vi "Begin.vi"() -> (0 "error out":errorcluster)   [LabVIEW 2011]
doc: "Called before other user functions, this VI is expected to open initial I/O refnums, load in file data, and do all program initialization. Notice that the <B>error out</B> terminal is simply used for data flow. Wiring it to other structures or subVIs ensures that this VI runs first."
uses:
  <vilib>/Rock Robotics/WPI/Joystick/WPI_JoystickDeviceEnum.ctl
  <vilib>/Rock Robotics/SystemInterfaces/DIO/FPGA_DIOPWMChannel.ctl
  <vilib>/Rock Robotics/SystemInterfaces/DIO/FPGA_DIOChannel.ctl
  <vilib>/Rock Robotics/SystemInterfaces/AI/FPGA_AIChannel.ctl
  <vilib>/Rock Robotics/SystemInterfaces/DIO/FPGA_DIORelayChannel.ctl
  <vilib>/Rock Robotics/SystemInterfaces/Typedef/FPGA_TypedefDigitalModule.ctl
  <vilib>/Rock Robotics/WPI/Relay/WPI_RelayDirection.ctl
  <vilib>/Rock Robotics/SystemInterfaces/AI/FPGA_AIGyroChannel.ctl
  <vilib>/Rock Robotics/WPI/RobotDrive/WPI_RobotDriveOpen4MotorWithJaguar.vi
  <vilib>/Rock Robotics/WPI/MotorControl/WPI_MotorControlOpen Victor.vi
  <vilib>/Rock Robotics/WPI/MotorControl/WPI_MotorControlOpen Jaguar.vi
  <vilib>/Rock Robotics/WPI/Counter/WPI_CounterDigitalInputToDigitalSource.vi
  <vilib>/Rock Robotics/WPI/Encoder/WPI_EncoderType.ctl
  <vilib>/Rock Robotics/WPI/MotorControl/WPI_MotorControlOpenCANJaguar.vi
  <vilib>/Rock Robotics/WPI/CAN/Jaguar/SubVIs/WPI_CANJaguar_ControlMode.ctl
  <vilib>/Rock Robotics/WPI/CAN/Jaguar/SubVIs/WPI_CANJaguar_SpeedReference.ctl
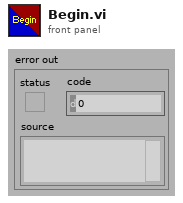
[diagram p1: front panel]
types:
  T1 = typedef "FPGA_AIChannel.ctl" = enum8{"AI 1", "AI 2", "AI 3", "AI 4", "AI 5", "AI 6", "AI 7", "AI 8", "Invalid"}
  T2 = typedef "WPI_JoystickDeviceEnum.ctl" = enum16{"USB 1", "USB 2", "USB 3", "USB 4", "Kinect 1", "Kinect 2"}
  T3 = typedef "FPGA_DIOChannel.ctl" = enum8{"DIO 1", "DIO 2", "DIO 3", "DIO 4", "DIO 5", "DIO 6", "DIO 7", "DIO 8", "DIO 9", "DIO 10", "DIO 11", "DIO 12", "DIO 13", "DIO 14", "Invalid"}
  T4 = typedef "FPGA_DIOPWMChannel.ctl" = enum8{"PWM 1", "PWM 2", "PWM 3", "PWM 4", "PWM 5", "PWM 6", "PWM 7", "PWM 8", "PWM 9", "PWM 10", "Invalid"}
  T5 = typedef "FPGA_AIGyroChannel.ctl" = enum8{"AI 1", "AI 2", "Invalid"}
  T6 = typedef "WPI_GyroDevRef.ctl" = cluster{"DevStatus":errorcluster, "Analog Module":T7, "Analog Channel":T1, "Offset":dbl, "Gain (VoltsPerDegree/Second)":dbl}
  T7 = typedef "FPGA_TypedefAnalogModule.ctl" = enum16{"Analog Module 1", "Analog Module 2"}
  T8 = typedef "FPGA_TypedefDigitalModule.ctl" = enum16{"Digital Module 1", "Digital Module 2"}
  T9 = typedef "WPI_CANJaguar_ControlMode.ctl" = enum8{"Percent VBus", "Current", "Speed", "Position", "Voltage"}
  T10 = typedef "WPI_MotorControlDeviceRef.ctl" = cluster{"DeviceStatus":errorcluster, "Type":enum16{"PWM", "CAN"}, "PWM":cluster{"Digital Module":T8, "PWM Channel":T4, "DeadBand":T11}, "CAN":cluster{"Device Number":u8, "Control Mode":T9, "Semaphore":T12, "Max Vout":dbl}, "Invert":bool, "TransformRef":T13, "InvTransformRef":T13}
  T11 = typedef "WPI_PWMDeadband.ctl" = cluster{"Name":string, "maxPositivePwm":i32, "minPositivePwm":i32, "centerPwm":i32, "maxNegativePwm":i32, "minNegativePwm":i32, "angularRange":u16}
  T12 = typedef "Semaphore RefNum" = refnum<k1>
  T13 = typedef "WPI_PWMTransform_ConPane.ctl" = refnum<vi>
  T14 = typedef "WPI_CANJaguar_SpeedReference.ctl" = u8
  T15 = typedef "WPI_DigitalInputDevRef.ctl" = cluster{"DevStatus":errorcluster, "DIO Channel":T3, "Digital Module":T8}
  T16 = typedef "WPI_EncoderType.ctl" = enum16{"1x", "2x", "4x"}
  T17 = typedef "FPGA_CounterEncoderSourceConvertionLVSourceType.ctl" = cluster{"DevStatus":errorcluster, "AnalogTriggerMode?":bool, "DigitalMode":cluster{"Digital Module":T8, "DIO Channel":T18}, "AnalogTriggerMode":cluster{"AnalogTriggerIndex":T19, "OutputType":T20}}
  T18 = typedef "FPGA_DIODigitalSourceChannel.ctl" = enum8{"DIO 1", "DIO 2", "DIO 3", "DIO 4", "DIO 5", "DIO 6", "DIO 7", "DIO 8", "DIO 9", "DIO 10", "DIO 11", "DIO 12", "DIO 13", "DIO 14", "Disabled"}
  T19 = typedef "FPGA_AnalogTriggerIndex.ctl" = enum8{"Trig 0", "Trig 1", "Trig 2", "Trig 3", "Trig 4", "Trig 5", "Trig 6", "Trig 7", "Invalid"}
  T20 = typedef "FPGA_AnalogTriggerOutType.ctl" = enum16{"InWindow", "TriggerState", "Rising", "Falling"}
  T21 = typedef "WPI_EncoderDevRef.ctl" = cluster{"DevStatus":errorcluster, "EncoderIndex":T22, "CounterIndex":T23, "DistancePerCount":dbl, "Decoding Type":T16}
  T22 = typedef "FPGA_EncoderIdx.ctl" = enum8{"Enc 0", "Enc 1", "Enc 2", "Enc 3", "Invalid"}
  T23 = typedef "FPGA_CounterCtrSystemIndex.ctl" = enum8{"Ctr 0", "Ctr 1", "Ctr 2", "Ctr 3", "Ctr 4", "Ctr 5", "Ctr 6", "Ctr 7", "Invalid"}
  T24 = typedef "WPI_ServoDeviceRef.ctl" = cluster{"DeviceStatus":errorcluster, "Digital Module":T8, "PWM Channel":T4, "DeadBand":T11}
  T25 = typedef "FPGA_DIORelayChannel.ctl" = enum8{"Relay 1", "Relay 2", "Relay 3", "Relay 4", "Relay 5", "Relay 6", "Relay 7", "Relay 8", "Invalid"}
  T26 = typedef "WPI_RelayDirection.ctl" = enum16{"Both directions", "Forward only", "Reverse only"}
  T27 = typedef "WPI_RelayDevRef.ctl" = cluster{"DevStatus":errorcluster, "Relay Channel":T25, "Digital Module":T8, "Relay Direction":T26}
  T28 = typedef "WPI_RobotDriveDevRef.ctl" = cluster{"DevStatus":errorcluster, "Motors[]":T10[], "Square Inputs":bool, "Max Output":dbl, "Isochronous":bool}
  T29 = typedef "WPI_JoystickDevRef.ctl" = cluster{"Device":T2}
  T30 = typedef "WPI_AnalogChannelDevRef.ctl" = cluster{"DevStatus":errorcluster, "Analog Module":T7, "Analog Channel":T1}
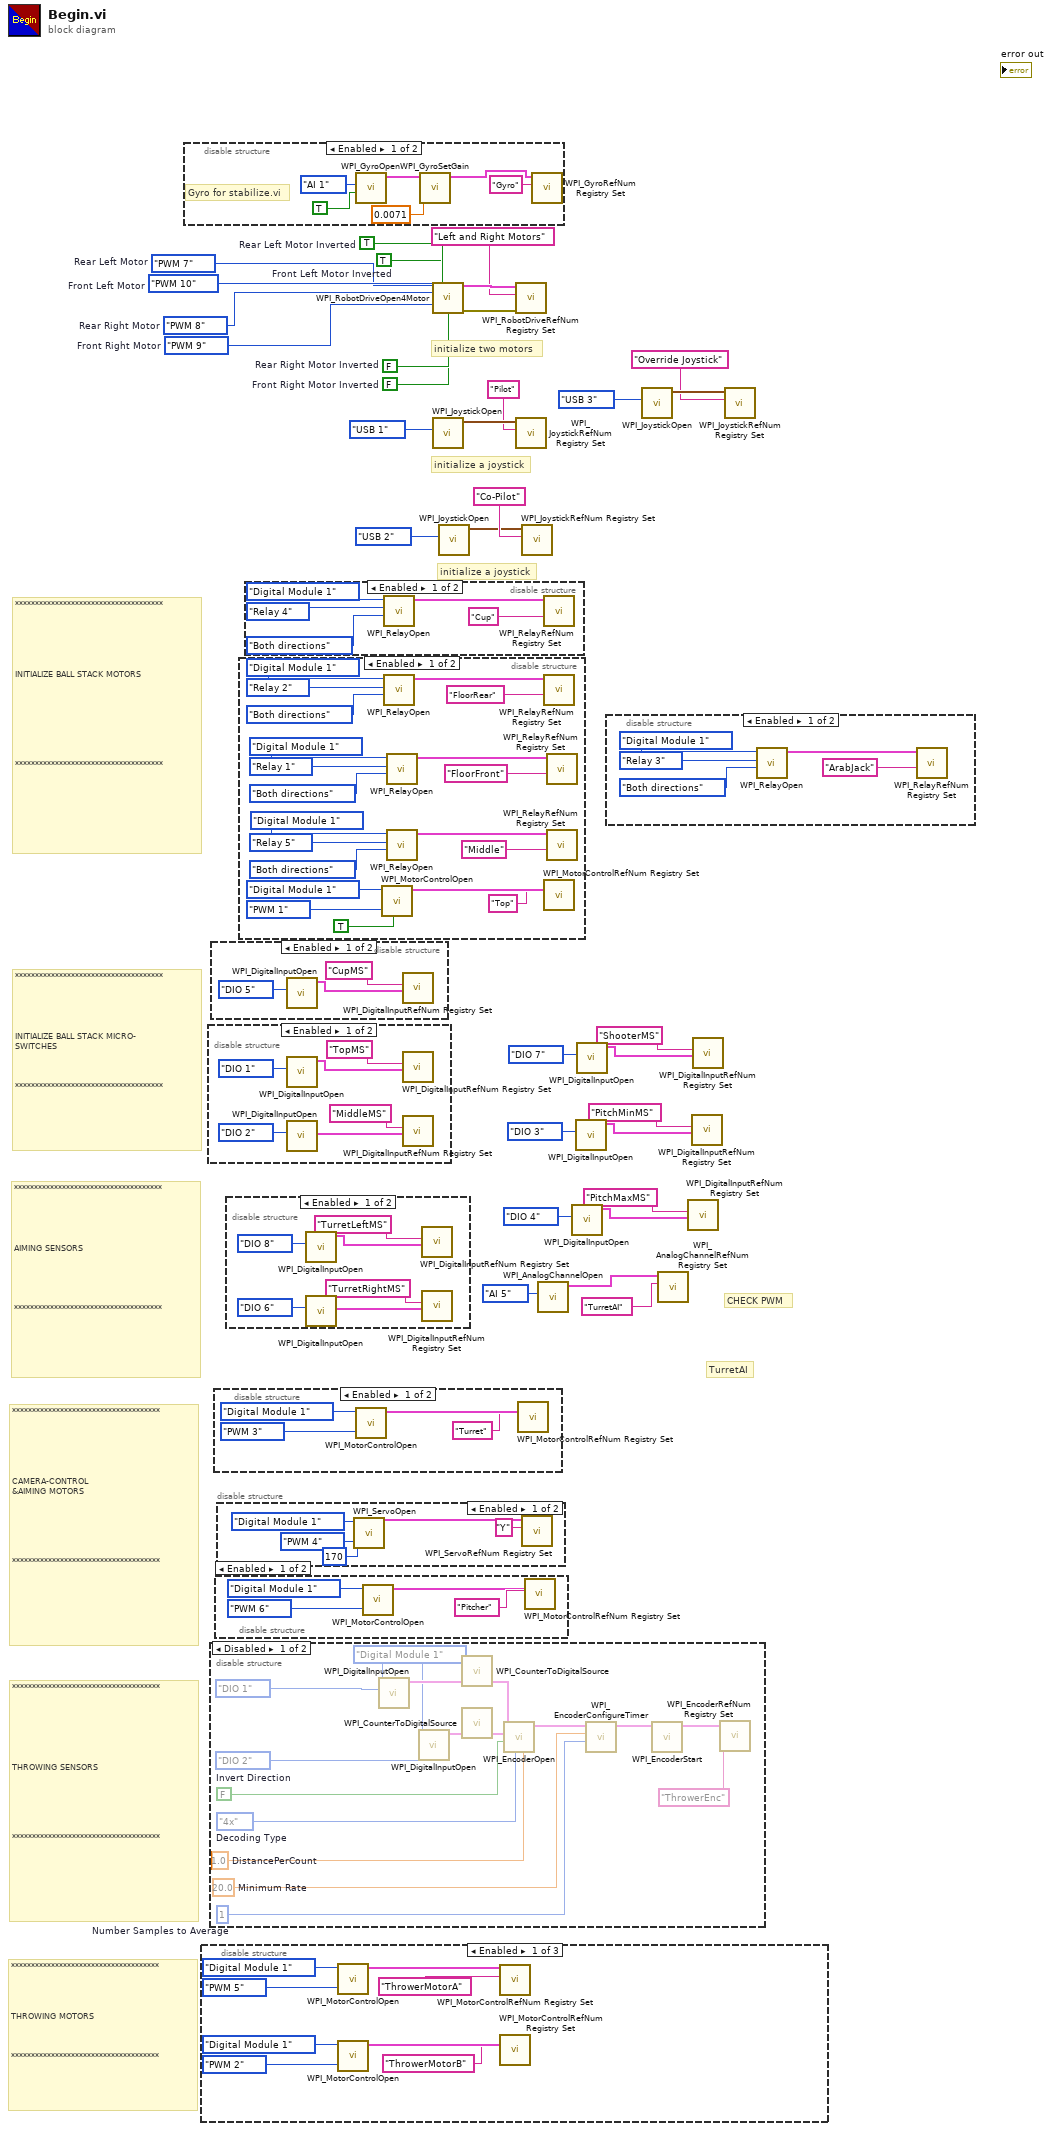
[diagram p0: block diagram]
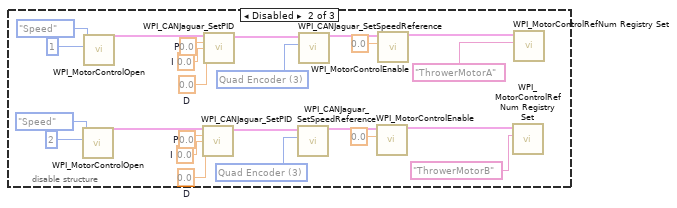
[diagram p13: hidden frame]
diagram:
  w16 = FALSE  # Front Right Motor Inverted
  w17 = TRUE  # Front Left Motor Inverted
  w18 = FPGA_DIOPWMChannel."PWM 7"  # Rear Left Motor
  w19 = FPGA_DIOPWMChannel."PWM 8"  # Rear Right Motor
  w20 = FPGA_DIOPWMChannel."PWM 9"  # Front Right Motor
  w21 = FPGA_DIOPWMChannel."PWM 10"  # Front Left Motor
  w31 = TRUE  # Rear Left Motor Inverted
  w32 = FALSE  # Rear Right Motor Inverted
  # "CHECK PWM"
  # "TurretAI"
  # "*************************************\n\n\n\n\nTHROWING MOTORS\n\n\n\n*************************************"
  # "*************************************\n\n\n\n\n\n\n\nTHROWING SENSORS\n\n\n\n\n\n\n*************************************"
  # "*************************************\n\n\n\n\n\n\nCAMERA-CONTROL\n&AIMING MOTORS\n\n\n\n\n\n\n*************************************"
  # "*************************************\n\n\n\n\n\nAIMING SENSORS\n\n\n\n\n\n*************************************"
  # "*************************************\n\n\n\n\n\nINITIALIZE BALL STACK MICRO-\nSWITCHES\n\n\n\n*************************************"
  # "*************************************\n\n\n\n\n\n\nINITIALIZE BALL STACK MOTORS\n\n\n\n\n\n\n\n\n*************************************"
  # "initialize a joystick"
  # "initialize a joystick"
  # "initialize two motors"
  n1 = disable-structure shown="Enabled" {
    frame Enabled {
      # "Gyro for stabilize.vi"
      n2 = call <vilib>:"WPI_GyroOpen.vi"("Calibrate On Open"=TRUE, "Analog Channel"=FPGA_AIGyroChannel."AI 1") -> ("GyroDevRef"=w35:T6)  [unwired: 7 in, 2 out]
      n3 = call <vilib>:"WPI_GyroSetGain.vi"("Gain (VoltsPerDegree/Second)"=0.0071, "GyroDevRef"=w35) -> ("GyroDevRef"=w34:T6)  [unwired: 1 in, 8 out]
      n4 = call <vilib>:"WPI_GyroRefNum Registry Set.vi"("refnum name"="Gyro", "GyroDevRef"=w34) -> ()  [unwired: 8 in, 2 out]
    }
    frame Disabled {
    }
  }
  n5 = disable-structure shown="Enabled" {
    frame Enabled {
      n6 = call-poly <vilib>:"WPI_MotorControlOpen.vi"("PWM Channel"=FPGA_DIOPWMChannel."PWM 5", "Digital Module (Module 1)"=FPGA_TypedefDigitalModule."Digital Module 1") -> ("MotorControlDeviceRef"=w46:T10)  [unwired: 8 in, 1 out]
      n7 = call-poly <vilib>:"WPI_MotorControlOpen.vi"("PWM Channel"=FPGA_DIOPWMChannel."PWM 2", "Digital Module (Module 1)"=FPGA_TypedefDigitalModule."Digital Module 1") -> ("MotorControlDeviceRef"=w42:T10)  [unwired: 8 in, 1 out]
      n8 = call <vilib>:"WPI_MotorControlRefNum Registry Set.vi"("refnum name"="ThrowerMotorA", "MotorControlDevRef"=w46) -> ()  [unwired: 8 in, 2 out]
      n9 = call <vilib>:"WPI_MotorControlRefNum Registry Set.vi"("refnum name"="ThrowerMotorB", "MotorControlDevRef"=w42) -> ()  [unwired: 8 in, 2 out]
    }
    frame Disabled {
      w59 = 0.0  # D
      w58 = 0.0  # I
      w57 = 0.0  # P
      w54 = T14 3 items=["Encoder"=0, "Inv Encoder"=2, "Quad Encoder"=3, "None"=255] ("Speed Reference")
      w60 = 0.0  # D
      w61 = 0.0  # I
      w62 = 0.0  # P
      w65 = T14 3 items=["Encoder"=0, "Inv Encoder"=2, "Quad Encoder"=3, "None"=255] ("Speed Reference")
      n10 = call-poly <vilib>:"WPI_MotorControlOpen.vi"("Device Number"=u8 2, "Control Mode"=WPI_CANJaguar_ControlMode."Speed") -> ("MotorControlDeviceRef"=w55:T10)  [unwired: 8 in, 1 out]
      n11 = call-poly <vilib>:"WPI_MotorControlOpen.vi"("Device Number"=u8 1, "Control Mode"=WPI_CANJaguar_ControlMode."Speed") -> ("MotorControlDeviceRef"=w64:T10)  [unwired: 8 in, 1 out]
      n12 = call <vilib>:"WPI_CANJaguar_SetPID.vi"("CAN Jaguar Ref"=w55, "P"=w57, "I"=w58, "D"=w59) -> ("CAN Jaguar Ref Out"=w53:T10)  [unwired: 10 in, 1 out]
      n13 = call <vilib>:"WPI_CANJaguar_SetPID.vi"("CAN Jaguar Ref"=w64, "P"=w62, "I"=w61, "D"=w60) -> ("CAN Jaguar Ref Out"=w66:T10)  [unwired: 10 in, 1 out]
      n14 = call <vilib>:"WPI_CANJaguar_SetSpeedReference.vi"("Speed Reference"=w54, "CAN Jaguar Ref"=w53) -> ("CAN Jaguar Ref Out"=w51:T10)  [unwired: 8 in, 1 out]
      n15 = call <vilib>:"WPI_CANJaguar_SetSpeedReference.vi"("Speed Reference"=w65, "CAN Jaguar Ref"=w66) -> ("CAN Jaguar Ref Out"=w68:T10)  [unwired: 8 in, 1 out]
      n16 = call <vilib>:"WPI_MotorControlEnable.vi"("Encoder Initial Position"=0.0, "CAN Jaguar Ref"=w51) -> ("CAN Jaguar Ref Out"=w50:T10)  [unwired: 8 in, 1 out]
      n17 = call <vilib>:"WPI_MotorControlEnable.vi"("Encoder Initial Position"=0.0, "CAN Jaguar Ref"=w68) -> ("CAN Jaguar Ref Out"=w69:T10)  [unwired: 8 in, 1 out]
      n18 = call <vilib>:"WPI_MotorControlRefNum Registry Set.vi"("refnum name"="ThrowerMotorB", "MotorControlDevRef"=w50) -> ()  [unwired: 8 in, 2 out]
      n19 = call <vilib>:"WPI_MotorControlRefNum Registry Set.vi"("refnum name"="ThrowerMotorA", "MotorControlDevRef"=w69) -> ()  [unwired: 8 in, 2 out]
    }
    frame Disabled {
    }
  }
  n20 = disable-structure shown="Enabled" {
    frame Enabled {
      n21 = call <vilib>:"WPI_DigitalInputOpen.vi"("DIO Channel"=FPGA_DIOChannel."DIO 1") -> ("DigitalInputDevRef"=w71:T15)  [unwired: 9 in, 1 out]
      n22 = call <vilib>:"WPI_DigitalInputOpen.vi"("DIO Channel"=FPGA_DIOChannel."DIO 2") -> ("DigitalInputDevRef"=w74:T15)  [unwired: 9 in, 1 out]
      n23 = call <vilib>:"WPI_DigitalInputRefNum Registry Set.vi"("refnum name"="TopMS", "DigitalInputDevRef"=w71) -> ()  [unwired: 8 in, 2 out]
      n24 = call <vilib>:"WPI_DigitalInputRefNum Registry Set.vi"("refnum name"="MiddleMS", "DigitalInputDevRef"=w74) -> ()  [unwired: 8 in, 2 out]
    }
    frame Disabled {
    }
  }
  n25 = disable-structure shown="Disabled" {
    frame Disabled {
      w80 = u8 1  # Number Samples to Average
      w81 = 20.0  # Minimum Rate
      w86 = 1.0  # DistancePerCount
      w85 = WPI_EncoderType."4x"  # Decoding Type
      w84 = FALSE  # Invert Direction
      w79 = FPGA_TypedefDigitalModule."Digital Module 1" ("DIO Module")
      n26 = call <vilib>:"WPI_DigitalInputOpen.vi"("DIO Channel"=FPGA_DIOChannel."DIO 1" ("A Channel"), "Digital Module (Module 1)"=w79) -> ("DigitalInputDevRef"=w90:T15)  [unwired: 1 in, 8 out]
      n27 = call <vilib>:"WPI_DigitalInputOpen.vi"("DIO Channel"=FPGA_DIOChannel."DIO 2" ("B Channel"), "Digital Module (Module 1)"=w79) -> ("DigitalInputDevRef"=w91:T15)  [unwired: 1 in, 8 out]
      n28 = call-poly <vilib>:"WPI_CounterToDigitalSource.vi"("DigitalInputDevRef"=w90) -> ("Digital Source"=w89:T17)  [unwired: 6 out]
      n29 = call-poly <vilib>:"WPI_CounterToDigitalSource.vi"("DigitalInputDevRef"=w91) -> ("Digital Source"=w92:T17)  [unwired: 6 out]
      n30 = call <vilib>:"WPI_EncoderOpen.vi"("DistancePerCount"=w86, "Decoding Type"=w85, "Invert Direction (False)"=w84, "BSource"=w92, "ASource"=w89) -> ("EncoderDevRef"=w82:T21)  [unwired: 3 in, 3 out]
      n31 = call <vilib>:"WPI_EncoderConfigureTimer.vi"("Number Samples to Average"=w80, "Minimum Rate"=w81, "EncoderDevRef"=w82) -> ("EncoderDevRef"=w83:T21)  [unwired: 1 in, 7 out]
      n32 = call <vilib>:"WPI_EncoderStart.vi"("EncoderDevRef"=w83) -> ("EncoderDevRef"=w78:T21)  [unwired: 1 in, 9 out]
      n33 = call <vilib>:"WPI_EncoderRefNum Registry Set.vi"("refnum name"="ThrowerEnc", "EncoderDevRef"=w78) -> ()  [unwired: 8 in, 2 out]
    }
    frame Enabled {
    }
  }
  n34 = disable-structure shown="Enabled" {
    frame Enabled {
      n35 = call <vilib>:"WPI_DigitalInputOpen.vi"("DIO Channel"=FPGA_DIOChannel."DIO 5") -> ("DigitalInputDevRef"=w95:T15)  [unwired: 9 in, 1 out]
      n36 = call <vilib>:"WPI_DigitalInputRefNum Registry Set.vi"("refnum name"="CupMS", "DigitalInputDevRef"=w95) -> ()  [unwired: 8 in, 2 out]
    }
    frame Disabled {
    }
  }
  n37 = disable-structure shown="Enabled" {
    frame Enabled {
      n38 = call-poly <vilib>:"WPI_MotorControlOpen.vi"("PWM Channel"=FPGA_DIOPWMChannel."PWM 3", "Digital Module (Module 1)"=FPGA_TypedefDigitalModule."Digital Module 1") -> ("MotorControlDeviceRef"=w99:T10)  [unwired: 8 in, 1 out]
      n39 = call <vilib>:"WPI_MotorControlRefNum Registry Set.vi"("refnum name"="Turret", "MotorControlDevRef"=w99) -> ()  [unwired: 8 in, 2 out]
    }
    frame Disabled {
    }
  }
  n40 = disable-structure shown="Enabled" {
    frame Enabled {
      n41 = call-poly <vilib>:"WPI_MotorControlOpen.vi"("PWM Channel"=FPGA_DIOPWMChannel."PWM 6", "Digital Module (Module 1)"=FPGA_TypedefDigitalModule."Digital Module 1") -> ("MotorControlDeviceRef"=w100:T10)  [unwired: 8 in, 1 out]
      n42 = call <vilib>:"WPI_MotorControlRefNum Registry Set.vi"("refnum name"="Pitcher", "MotorControlDevRef"=w100) -> ()  [unwired: 8 in, 2 out]
    }
    frame Disabled {
    }
  }
  n43 = disable-structure shown="Enabled" {
    frame Enabled {
      n44 = call <vilib>:"WPI_ServoOpen.vi"("Angular Range"=u16 170, "PWM Channel"=FPGA_DIOPWMChannel."PWM 4", "Digital Module (Module 1)"=FPGA_TypedefDigitalModule."Digital Module 1") -> ("ServoDeviceRef"=w105:T24)  [unwired: 7 in, 1 out]
      n45 = call <vilib>:"WPI_ServoRefNum Registry Set.vi"("refnum name"="Y", "ServoDeviceRef"=w105) -> ()  [unwired: 8 in, 2 out]
    }
    frame Disabled {
    }
  }
  n46 = disable-structure shown="Enabled" {
    frame Enabled {
      n47 = call <vilib>:"WPI_DigitalInputOpen.vi"("DIO Channel"=FPGA_DIOChannel."DIO 8") -> ("DigitalInputDevRef"=w109:T15)  [unwired: 9 in, 1 out]
      n48 = call <vilib>:"WPI_DigitalInputOpen.vi"("DIO Channel"=FPGA_DIOChannel."DIO 6") -> ("DigitalInputDevRef"=w112:T15)  [unwired: 9 in, 1 out]
      n49 = call <vilib>:"WPI_DigitalInputRefNum Registry Set.vi"("refnum name"="TurretLeftMS", "DigitalInputDevRef"=w109) -> ()  [unwired: 8 in, 2 out]
      n50 = call <vilib>:"WPI_DigitalInputRefNum Registry Set.vi"("refnum name"="TurretRightMS", "DigitalInputDevRef"=w112) -> ()  [unwired: 8 in, 2 out]
    }
    frame Disabled {
    }
  }
  n51 = disable-structure shown="Enabled" {
    frame Enabled {
      n52 = call-poly <vilib>:"WPI_MotorControlOpen.vi"("Invert"=TRUE, "PWM Channel"=FPGA_DIOPWMChannel."PWM 1", "Digital Module (Module 1)"=FPGA_TypedefDigitalModule."Digital Module 1") -> ("MotorControlDeviceRef"=w129:T10)  [unwired: 7 in, 1 out]
      n53 = call <vilib>:"WPI_RelayOpen.vi"("Relay Direction"=WPI_RelayDirection."Both directions", "Relay Channel"=FPGA_DIORelayChannel."Relay 2", "Digital Module (Module 1)"=FPGA_TypedefDigitalModule."Digital Module 1") -> ("RelayDevRef"=w131:T27)  [unwired: 7 in, 1 out]
      n54 = call <vilib>:"WPI_RelayOpen.vi"("Relay Direction"=WPI_RelayDirection."Both directions", "Relay Channel"=FPGA_DIORelayChannel."Relay 1", "Digital Module (Module 1)"=FPGA_TypedefDigitalModule."Digital Module 1") -> ("RelayDevRef"=w119:T27)  [unwired: 7 in, 1 out]
      n55 = call <vilib>:"WPI_RelayOpen.vi"("Relay Direction"=WPI_RelayDirection."Both directions", "Relay Channel"=FPGA_DIORelayChannel."Relay 5", "Digital Module (Module 1)"=FPGA_TypedefDigitalModule."Digital Module 1") -> ("RelayDevRef"=w122:T27)  [unwired: 7 in, 1 out]
      n56 = call <vilib>:"WPI_RelayRefNum Registry Set.vi"("refnum name"="FloorRear", "RelayDevRef"=w131) -> ()  [unwired: 8 in, 2 out]
      n57 = call <vilib>:"WPI_MotorControlRefNum Registry Set.vi"("refnum name"="Top", "MotorControlDevRef"=w129) -> ()  [unwired: 8 in, 2 out]
      n58 = call <vilib>:"WPI_RelayRefNum Registry Set.vi"("refnum name"="FloorFront", "RelayDevRef"=w119) -> ()  [unwired: 8 in, 2 out]
      n59 = call <vilib>:"WPI_RelayRefNum Registry Set.vi"("refnum name"="Middle", "RelayDevRef"=w122) -> ()  [unwired: 8 in, 2 out]
    }
    frame Disabled {
    }
  }
  n60 = disable-structure shown="Enabled" {
    frame Enabled {
      n61 = call <vilib>:"WPI_RelayOpen.vi"("Relay Direction"=WPI_RelayDirection."Both directions", "Relay Channel"=FPGA_DIORelayChannel."Relay 4", "Digital Module (Module 1)"=FPGA_TypedefDigitalModule."Digital Module 1") -> ("RelayDevRef"=w138:T27)  [unwired: 7 in, 1 out]
      n62 = call <vilib>:"WPI_RelayRefNum Registry Set.vi"("refnum name"="Cup", "RelayDevRef"=w138) -> ()  [unwired: 8 in, 2 out]
    }
    frame Disabled {
    }
  }
  n63 = call-poly <vilib>:"WPI_RobotDriveOpen4Motor.vi"("Rear Left Motor"=w18, "Rear Left Motor Inverted"=w31, "Rear Right Motor Inverted"=w32, "Rear Right Motor"=w19, "Front Left Motor"=w21, "Front Right Motor"=w20, "Front Left Motor Inverted"=w17, "Front Right Motor Inverted"=w16) -> ("RobotDriveDevRef"=w30:T28, "error out"=w26:errorcluster)  [unwired: 6 in]
  n64 = call <vilib>:"WPI_JoystickOpen.vi"("JoystickDevice"=WPI_JoystickDeviceEnum."USB 1") -> ("JoystickDevRef"=w28:T29)  [unwired: 10 out]
  n65 = call <vilib>:"WPI_JoystickOpen.vi"("JoystickDevice"=WPI_JoystickDeviceEnum."USB 2") -> ("JoystickDevRef"=w22:T29)  [unwired: 10 out]
  n66 = call <vilib>:"WPI_RobotDriveRefNum Registry Set.vi"("error in (no error)"=w26, "refnum name"="Left and Right Motors", "RobotDriveDevRef"=w30) -> ()  [unwired: 9 out]
  n67 = call <vilib>:"WPI_JoystickRefNum Registry Set.vi"("refnum name"="Pilot", "JoystickDevRef"=w28) -> ()  [unwired: 1 in, 9 out]
  n68 = call <vilib>:"WPI_JoystickRefNum Registry Set.vi"("refnum name"="Co-Pilot", "JoystickDevRef"=w22) -> ()  [unwired: 1 in, 9 out]
  n69 = call <vilib>:"WPI_AnalogChannelOpen.vi"("Analog Channel"=FPGA_AIChannel."AI 5") -> ("AIDeviceRef"=w2:T30)  [unwired: 9 in, 1 out]
  n70 = call <vilib>:"WPI_DigitalInputOpen.vi"("DIO Channel"=FPGA_DIOChannel."DIO 4") -> ("DigitalInputDevRef"=w13:T15)  [unwired: 9 in, 1 out]
  n71 = call <vilib>:"WPI_DigitalInputOpen.vi"("DIO Channel"=FPGA_DIOChannel."DIO 3") -> ("DigitalInputDevRef"=w12:T15)  [unwired: 9 in, 1 out]
  n72 = call <vilib>:"WPI_DigitalInputOpen.vi"("DIO Channel"=FPGA_DIOChannel."DIO 7") -> ("DigitalInputDevRef"=w7:T15)  [unwired: 9 in, 1 out]
  n73 = disable-structure shown="Enabled" {
    frame Enabled {
      n74 = call <vilib>:"WPI_RelayOpen.vi"("Relay Direction"=WPI_RelayDirection."Both directions", "Relay Channel"=FPGA_DIORelayChannel."Relay 3", "Digital Module (Module 1)"=FPGA_TypedefDigitalModule."Digital Module 1") -> ("RelayDevRef"=w141:T27)  [unwired: 7 in, 1 out]
      n75 = call <vilib>:"WPI_RelayRefNum Registry Set.vi"("refnum name"="ArabJack", "RelayDevRef"=w141) -> ()  [unwired: 8 in, 2 out]
    }
    frame Disabled {
    }
  }
  n76 = call <vilib>:"WPI_JoystickOpen.vi"("JoystickDevice"=WPI_JoystickDeviceEnum."USB 3") -> ("JoystickDevRef"=w6:T29)  [unwired: 10 out]
  n77 = call <vilib>:"WPI_AnalogChannelRefNum Registry Set.vi"("refnum name"="TurretAI", "AIDeviceRef"=w2) -> ()  [unwired: 8 in, 2 out]
  n78 = call <vilib>:"WPI_DigitalInputRefNum Registry Set.vi"("refnum name"="PitchMaxMS", "DigitalInputDevRef"=w13) -> ()  [unwired: 8 in, 2 out]
  n79 = call <vilib>:"WPI_DigitalInputRefNum Registry Set.vi"("refnum name"="PitchMinMS", "DigitalInputDevRef"=w12) -> ()  [unwired: 8 in, 2 out]
  n80 = call <vilib>:"WPI_DigitalInputRefNum Registry Set.vi"("refnum name"="ShooterMS", "DigitalInputDevRef"=w7) -> ()  [unwired: 8 in, 2 out]
  n81 = call <vilib>:"WPI_JoystickRefNum Registry Set.vi"("refnum name"="Override Joystick", "JoystickDevRef"=w6) -> ()  [unwired: 1 in, 9 out]
